vi "INTELLIFAUCET Initialize MW100.vi"(4 "Refnum in":T1, 6 "Debug":bool, 8 "error in (no error)":errorcluster, 11 "MW100 Input":refnum<visa-resource-name>) -> (0 "error out":errorcluster, 2 "Local?":bool, 3 "MW100 Output":refnum<visa-resource-name>)   [LabVIEW 2016]
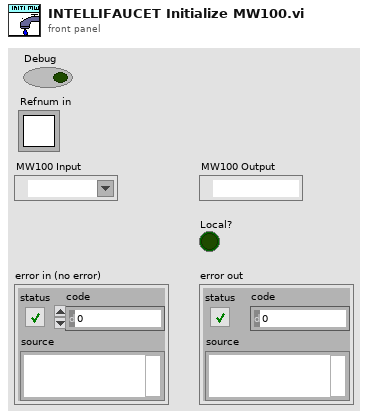
[diagram p1: front panel]
types:
  T1 = typedef "Semaphore RefNum" = refnum<k1>
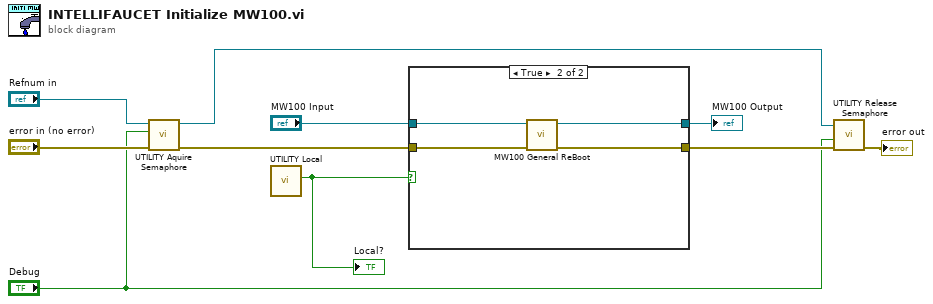
[diagram p0: block diagram]
diagram:
  n1 = call "UTILITY Aquire Semaphore.vi"("error in (no error)"="error in (no error)", "Debug"="Debug", "Refnum in"="Refnum in") -> ("error out"=w5:errorcluster, "Refnum out"=w4:T1)  [unwired: 6 in, 1 out]
  n2 = call "UTILITY Local.vi"() -> ("Local?"=w1:bool)  [unwired: 11 in]
  "Local?" <- w1
  n3 = case shown="True" w1 {
    tunnel: w5 -> [w12 w16]
    tunnel: [w12 w15] -> w7
    tunnel: "MW100 Input" -> [w11 w14]
    tunnel: [w11 w13] -> w10
    frame False {
    }
    frame True {
      n4 = call "MW100 General ReBoot.vi"("error in (no error)"=w16, "VISA Refnum in"=w14) -> ("error out"=w15:errorcluster, "VISA Refnum out"=w13:refnum<visa-resource-name>)  [unwired: 8 in]
    }
  }
  "MW100 Output" <- w10
  n5 = call "UTILITY Release Semaphore.vi"("error in (no error)"=w7, "Debug"="Debug", "Refnum in"=w4) -> ("error out"=→"error out":errorcluster)  [unwired: 8 in]
